vi "GetBranchNumber.vi"(6 "error in":errorcluster, 9 "Terminal in":refnum<class "Terminal.lvclass">) -> (0 "error out":errorcluster, 3 "Terminal out":refnum<class "Terminal.lvclass">, 4 "branch":i32, 5 "wire branched":bool)   [LabVIEW 2014, in "Terminal.lvclass"]
uses:
  Terminal.lvclass
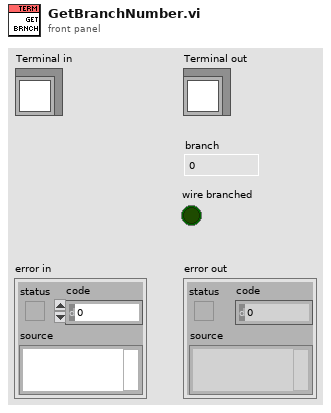
[diagram p1: front panel]
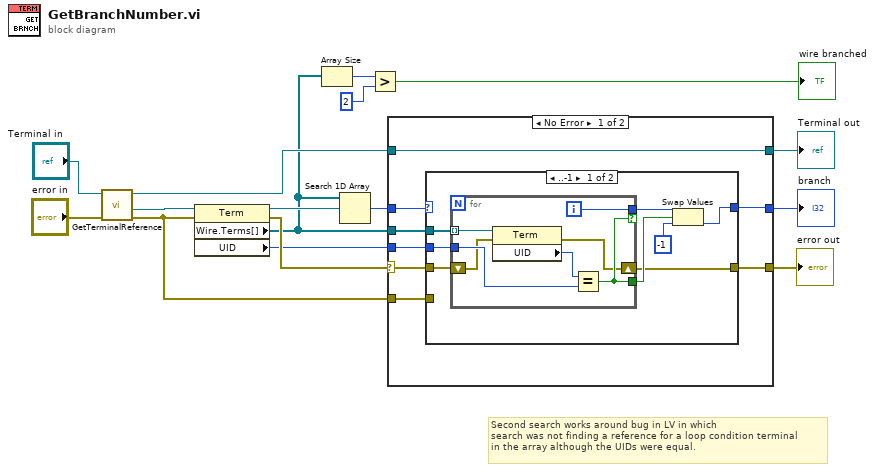
[diagram p0: block diagram]
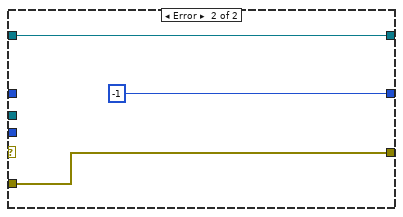
[diagram p3: hidden frame]
diagram:
  # "Second search works around bug in LV in which\nsearch was not finding a reference for a loop condition terminal\nin the array although the UIDs were equal."
  n1 = call "GetTerminalReference.vi"("error in"="error in", "Terminal in"="Terminal in") -> ("error out"=w13:errorcluster, "reference"=w14:refnum<vi>, "Terminal out"=w11:refnum<class "Terminal.lvclass">)  [unwired: 7 in]
  n2 = property class="Term"(reference=w14, error in=w13) -> (reference out=w8:refnum<vi>, error out=w9:errorcluster, "Wire.Terms[]"=w1:refnum<vi>[], "UID"=w2:i32)
  n3 = Array Size(array=w1) -> (size(s)=w6:i32)
  n4 = Search 1D Array(1D array=w1, element=w8) -> (index of element=w7:i32)  [unwired: 1 in]
  n5 = Greater?(x=w6, y=2) -> (0:→"wire branched":bool)
  n6 = case shown="No Error" w9 {
    selector: w9 -> [w20 _]
    tunnel: w13 -> [w22 w43]
    tunnel: [w24 w44] -> w12
    tunnel: w11 -> [w24 w44]
    tunnel: [w19 w43] -> w10
    tunnel: w7 -> [w23 _]
    tunnel: [w21 -1 ("index of element")] -> w3
    tunnel: w2 -> [w17 _]
    tunnel: w1 -> [w18 _]
    frame No Error {
      n7 = case shown="..-1" w23 {
        selector: w23 -> [_ w41]
        tunnel: w22 -> [_ _]
        tunnel: [w29 w41] -> w21
        tunnel: w20 -> [w26 w40]
        tunnel: [w25 w40] -> w19
        tunnel: w18 -> [w28 _]
        tunnel: w17 -> [w27 _]
        frame ..-1 {
          n8 = for {
            tunnel: w28 -> [w39] mode=indexing
            tunnel: [w38] -> w30 if=w36
            tunnel: [w36] -> w31
            tunnel: w27 -> [w35]
            shift-right: [w34] -> w25
            shift-left: w26 -> [w33]
            i -> [w38]
            n9 = property class="Term"(reference=w39, error in=w33) -> (error out=w34:errorcluster, "UID"=w37:i32)  [unwired: 1 out]
            n10 = Equal?(x=w37, y=w35) -> (x = y?=w36:bool)
          }
          n11 = Swap Values(12:w30, 13:w31, 14:-1 ("x")) -> (3:w29:i32)  [unwired: 1 out]
        }
        frame 0.. {
        }
      }
    }
    frame Error {
    }
  }
  "error out" <- w10
  "Terminal out" <- w12
  "branch" <- w3
